vi "Encoding.vi"(0 "transition_out":T1=3 items=["Disable_Voltage"=0, "Unknown"=3, "Quick_Stop"=2, "Shutdown"=6, "Enable_Operation"=15], 5 "halt":u16, 7 "Mode_out":i8(ring)=1 items=["Profile_Pos"=1, "Profile_Vel"=3, "Torque_Prof"=4, "Homing"=6, "Inter_Pos"=7], 9 "new_set_point":u16, 11 "reset":u16) -> (4 "controlword":u16, 6 "Outputs-mode_of_operation":i8)   [LabVIEW 2020]
uses:
  Controlword_transition.ctl
  ElementDTD.lvlib
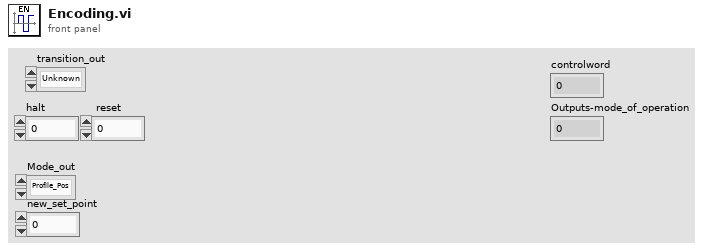
[diagram p1: front panel]
types:
  T1 = typedef "ElementDTD.lvlib/Controlword_transition.ctl" = u16
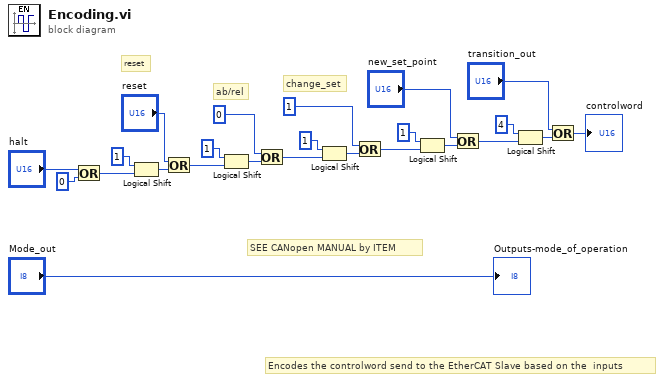
[diagram p0: block diagram]
diagram:
  # "SEE CANopen MANUAL by ITEM"
  # "Encodes the controlword send to the EtherCAT Slave based on the  inputs"
  # "change_set"
  # "ab/rel"
  # "reset"
  n1 = Or(x="halt", y=u16 0 ("Outputs-controlword")) -> (x .or. y?=w23:u16)
  n2 = Logical Shift(y=i16 1, x=w23) -> (x << y=w11:u16)
  n3 = Or(x="reset", y=w11) -> (x .or. y?=w21:u16)
  n4 = Logical Shift(y=i16 1, x=w21) -> (x << y=w10:u16)
  n5 = Or(x=u16 0, y=w10) -> (x .or. y?=w18:u16)
  n6 = Logical Shift(y=i16 1, x=w18) -> (x << y=w9:u16)
  n7 = Or(x=u16 1, y=w9) -> (x .or. y?=w15:u16)
  n8 = Logical Shift(y=i16 1, x=w15) -> (x << y=w8:u16)
  n9 = Or(x="new_set_point", y=w8) -> (x .or. y?=w13:u16)
  n10 = Logical Shift(y=i16 4, x=w13) -> (x << y=w7:u16)
  n11 = Or(x="transition_out", y=w7) -> (x .or. y?=→"controlword":T1)
  "Outputs-mode_of_operation" <- "Mode_out"
